vi "Create Alarm State Update Observer.vi"(8 "error in (no error)":errorcluster) -> (0 "error out":errorcluster, 3 "Alarm State":refnum<event-registration>)   [LabVIEW 2015, in "Alarm Handler Actor.lvclass"]
uses:
  Alarm Handler Actor.lvclass
  State.ctl
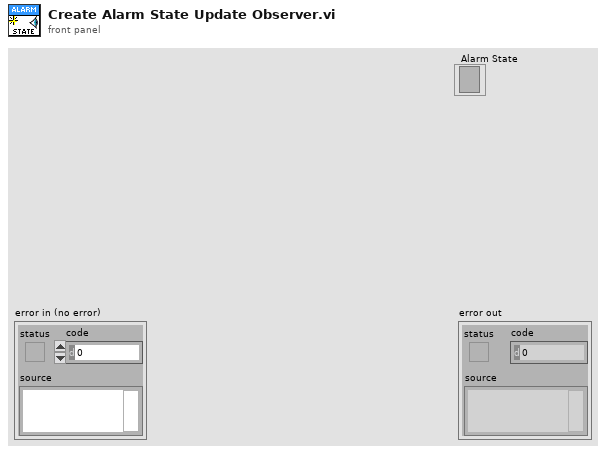
[diagram p1: front panel]
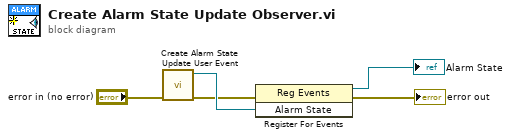
[diagram p0: block diagram]
diagram:
  n1 = call "Create Alarm State Update User Event.vi"("error in (no error)"="error in (no error)") -> ("error out"=w3:errorcluster, "Alarm State"=w4:refnum<user-event>)  [unwired: 9 in]
  n2 = register-events(error in=w3, w4) -> (reference out=→"Alarm State":refnum<event-registration>, error out=→"error out":errorcluster)  [unwired: 1 in]
